vi "IonGuide.vi"() -> ()   [LabVIEW 2014, in "Panels.lvlib"]
uses:
  Panels.lvlib
  CSlibraries-extern/DimLVEvent/DimIndicators/DimIndicators.lvlib
  CSlibraries/UtilityLib/UtilityLib.lvlib
  CS_Core/CSSystem/CoreLib/CoreLib.lvlib
  CSlibraries/UtilityLib/UtilityLib.valueStatus.ctl
  CSlibraries-extern/DimLVEvent/LVDimInterface/LVDimInterface.lvlib
  Instance           1 16Saved   IonGuide .vi
  CS_Core/CSSystem/CoreLib/CoreLib.double 2 byte array.vi
  CS_Core/CSSystem/CoreLib/CoreLib.string 2 byte array.vi
  CS_Core/CSSystem/CoreLib/CoreLib.short 2 byte array.vi
  CSlibraries-extern/DimLVEvent/DimIndicators/DimIndicators.numericType.ctl
  CS_Core/BaseProcess/BaseProcess.descriptor string definition.ctl
  CS_Core/BaseProcess/BaseProcess.lvlib
  CS_Core/CSSystem/CoreDefs/CoreDefs.rawDataType.ctl
  CS_Core/CSSystem/CoreDefs/CoreDefs.call_type.ctl
  CSlibraries-extern/DimLVEvent/DimIndicators/DimIndicators.numericArrayType.ctl
  CSlibraries-extern/DimLVEvent/DimIndicators/DimIndicators.anyType.ctl
panel:
  in  "ListOfBases_Data":T1={"data"="NOLINK", "no link"=TRUE, "quality"=-1, "timeStamp"=0.0}
  in  "DC8_SetValueInfoData":T2={"data"=[-118.7, 118.8, 3.0], "no link"=FALSE, "quality"=0, "timeStamp"=3265900746.569}
  in  "DC7_SetValueInfoData":T2={"data"=[-118.7, 118.8, 3.0], "no link"=FALSE, "quality"=0, "timeStamp"=3265900746.569}
  in  "DC6_SetValueInfoData":T2={"data"=[-118.7, 118.8, 3.0], "no link"=FALSE, "quality"=0, "timeStamp"=3265900746.569}
  in  "DC8_SetData":T2={"data"=[0.0, 0.0, 0.0, 0.0], "no link"=FALSE, "quality"=1, "timeStamp"=3265900745.1}
  in  "DC6_SetData":T2={"data"=[0.0, 0.0, 0.0, 0.0], "no link"=FALSE, "quality"=1, "timeStamp"=3265900745.335}
  in  "DC7_SetData":T2={"data"=[0.0, 0.0, 0.0, 0.0], "no link"=FALSE, "quality"=1, "timeStamp"=3265900745.1}
  in  "DC8":bool
  in  "DC6":bool
  in  "DC7":bool
  in  "Offset_SetValueInfoData":T2={"data"=[-400.0, 400.0, 3.0], "no link"=FALSE, "quality"=0, "timeStamp"=3265900746.522}
  in  "Mass_SetData":T2={"data"=[0.0, 0.0, 0.0, 0.0], "no link"=FALSE, "quality"=1, "timeStamp"=3265900745.1}
  in  "IonGuideBase_SetValueInfoData":T2={"data"=[-400.0, 400.0, 3.0], "no link"=FALSE, "quality"=0, "timeStamp"=3265900746.522}
  in  "SetFileLocation_Data":T1={"data"="NOLINK", "no link"=TRUE, "quality"=-1, "timeStamp"=0.0}
  out "error out":errorcluster
  out "vi reference":refnum<vi>
  in  "Alpha":bool
  out "Alpha_Mon":dbl=inf format="%.4f"
  in  "Offset":bool
  out "Offset_Mon":dbl=inf format="%.4f"
  in  "Mass":bool
  out "Mass_Mon":dbl=inf format="%.4f"
  in  "RFamp3":bool
  out "RFamp3_Mon":dbl=inf format="%.4f"
  in  "RFphase2":bool
  in  "RFphase1":bool
  in  "DC5":bool
  in  "DC4":bool
  in  "RFamp2":bool
  in  "uPlate2":bool
  in  "uDC1":bool
  in  "uDC2":bool
  in  "RFamp1":bool
  in  "IGADC2":bool
  in  "uPlate1":bool
  in  "IGADC3":bool
  in  "IGADC1":bool
  in  "Alpha_SetValueInfoData":T2={"data"=[-404.0, 401.8, 3.0], "no link"=FALSE, "quality"=0, "timeStamp"=3265900746.569}
  in  "Mass_SetValueInfoData":T2={"data"=[-404.0, 401.8, 3.0], "no link"=FALSE, "quality"=0, "timeStamp"=3265900746.569}
  in  "Offset_SetData":T2={"data"=[0.0, 0.0, 0.0, 0.0], "no link"=FALSE, "quality"=1, "timeStamp"=3265900745.053}
  in  "Alpha_SetData":T2={"data"=[0.0, 0.0, 0.0, 0.0], "no link"=FALSE, "quality"=1, "timeStamp"=3265900745.053}
  in  "Alpha_MonData":T3={"data"=inf, "no link"=FALSE, "quality"=1, "timeStamp"=3265900746.538}
  in  "Mass_MonData":T3={"data"=inf, "no link"=FALSE, "quality"=1, "timeStamp"=3265900746.569}
  in  "Offset_MonData":T3={"data"=inf, "no link"=FALSE, "quality"=1, "timeStamp"=3265900746.554}
  in  "DC5_SetValueInfoData":T2={"data"=[-400.0, 400.0, 3.0], "no link"=FALSE, "quality"=0, "timeStamp"=3265900746.522}
  in  "DC4_SetValueInfoData":T2={"data"=[-118.7, 118.8, 3.0], "no link"=FALSE, "quality"=0, "timeStamp"=3265900746.569}
  in  "uDC2_SetValueInfoData":T2={"data"=[-120.9, 120.5, 3.0], "no link"=FALSE, "quality"=0, "timeStamp"=3265900746.585}
  in  "uDC1_SetValueInfoData":T2={"data"=[-120.8, 120.3, 3.0], "no link"=FALSE, "quality"=0, "timeStamp"=3265900746.569}
  in  "RFamp3_SetData":T2={"data"=[0.0, 0.0, 0.0, 0.0], "no link"=FALSE, "quality"=1, "timeStamp"=3265900745.335}
  in  "RFphase2_SetData":T2={"data"=[0.0, 0.0, 0.0, 0.0], "no link"=FALSE, "quality"=1, "timeStamp"=3265900745.1}
  in  "RFphase1_SetData":T2={"data"=[0.0, 0.0, 0.0, 0.0], "no link"=FALSE, "quality"=1, "timeStamp"=3265900745.1}
  in  "DC5_SetData":T2={"data"=[0.0, 0.0, 0.0, 0.0], "no link"=FALSE, "quality"=1, "timeStamp"=3265900745.069}
  in  "DC8_MonData":T3={"data"=inf, "no link"=FALSE, "quality"=1, "timeStamp"=3265900746.538}
  in  "MFDC2_MonData":T3={"data"=inf, "no link"=FALSE, "quality"=1, "timeStamp"=3265900746.538}
  in  "MFDC1_MonData":T3={"data"=inf, "no link"=FALSE, "quality"=1, "timeStamp"=3265900746.522}
  in  "RFphase2_MonData":T3={"data"=inf, "no link"=FALSE, "quality"=1, "timeStamp"=3265900746.569}
  in  "RFphase1_MonData":T3={"data"=inf, "no link"=FALSE, "quality"=1, "timeStamp"=3265900746.554}
  in  "IGADC1_MonData":T3={"data"=inf, "no link"=FALSE, "quality"=1, "timeStamp"=3265900746.538}
  in  "RFamp1_MonData":T3={"data"=inf, "no link"=FALSE, "quality"=1, "timeStamp"=3265900746.569}
  in  "uPlate1_MonData":T3={"data"=inf, "no link"=FALSE, "quality"=1, "timeStamp"=3265900746.554}
  out "RFphase2_Mon":dbl=inf format="%.4f"
  out "RFphase1_Mon":dbl=inf format="%.4f"
  out "MFDC1_Mon":dbl=inf format="%.4f"
  out "MFDC2_Mon":dbl=inf format="%.4f"
  out "DC5_Mon":dbl=inf format="%.4f"
  out "DC7_Mon":dbl=inf format="%.4f"
  out "DC8_Mon":dbl=inf format="%.4f"
  out "DC6_Mon":dbl=inf format="%.4f"
  in  "uDC2_MonData":T3={"data"=inf, "no link"=FALSE, "quality"=1, "timeStamp"=3265900746.538}
  in  "IGADC2_MonData":T3={"data"=inf, "no link"=FALSE, "quality"=1, "timeStamp"=3265900746.569}
  out "IGBPEN_Mon":dbl=inf format="%.2e"
  out "IGCPEN_Mon":dbl=inf format="%.2e"
  in  "uPlate2_SetValueInfoData":T2={"data"=[-125.5, 126.0, 3.0], "no link"=FALSE, "quality"=0, "timeStamp"=3265900746.554}
  in  "DC4_SetData":T2={"data"=[0.0, 0.0, 0.0, 0.0], "no link"=FALSE, "quality"=1, "timeStamp"=3265900745.069}
  in  "RFamp2_SetValueInfoData":T2={"data"=[0.0, 400.0, -1.0], "no link"=FALSE, "quality"=0, "timeStamp"=3265900746.585}
  in  "uPlate2_SetData":T2={"data"=[0.0, 0.0, 0.0, 0.0], "no link"=FALSE, "quality"=1, "timeStamp"=3265900745.069}
  in  "DC7_MonData":T3={"data"=inf, "no link"=FALSE, "quality"=1, "timeStamp"=3265900746.569}
  out "RFamp1_Mon":dbl=inf format="%.4f"
  out "IGADC1_Mon":dbl=inf format="%.4f"
  out "i ref out":refnum<vi>
  in  "Last Loaded File_Data":T1={"data"="NOLINK", "no link"=TRUE, "quality"=-1, "timeStamp"=0.0}
  out "FileUpToDate":bool=TRUE caption="Parameter Changed"
  in  "Close All Panels":bool
  in  "IGADC1_SetValueInfoData":T2={"data"=[-401.3, 400.4, 3.0], "no link"=FALSE, "quality"=0, "timeStamp"=3265900746.554}
  in  "IGADC2_SetValueInfoData":T2={"data"=[-404.3, 403.0, 3.0], "no link"=FALSE, "quality"=0, "timeStamp"=3265900746.538}
  in  "IGADC3_SetValueInfoData":T2={"data"=[-400.3, 399.3, 3.0], "no link"=FALSE, "quality"=0, "timeStamp"=3265900746.569}
  in  "RFamp3_SetValueInfoData":T2={"data"=[0.0, 3000.0, -1.0], "no link"=FALSE, "quality"=0, "timeStamp"=3265900746.554}
  in  "RFphase1_SetValueInfoData":T2={"data"=[0.0, 10.0, -1.0], "no link"=FALSE, "quality"=0, "timeStamp"=3265900746.522}
  in  "RFphase2_SetValueInfoData":T2={"data"=[0.0, 10.0, -1.0], "no link"=FALSE, "quality"=0, "timeStamp"=3265900746.538}
  in  "RFamp1_SetValueInfoData":T2={"data"=[0.0, 1000.0, -1.0], "no link"=FALSE, "quality"=0, "timeStamp"=3265900746.538}
  in  "uPlate1_SetValueInfoData":T2={"data"=[-404.0, 401.8, 3.0], "no link"=FALSE, "quality"=0, "timeStamp"=3265900746.569}
  in  "IonGuideBase_SetData":T2={"data"=[0.0, 0.0, 0.0, 0.0], "no link"=FALSE, "quality"=1, "timeStamp"=3265900745.1}
  in  "uDC1_SetData":T2={"data"=[0.0, 0.0, 0.0, 0.0], "no link"=FALSE, "quality"=1, "timeStamp"=3265900745.069}
  in  "IGADC3_SetData":T2={"data"=[0.0, 0.0, 0.0, 0.0], "no link"=FALSE, "quality"=1, "timeStamp"=3265900745.053}
  in  "IGADC2_SetData":T2={"data"=[0.0, 0.0, 0.0, 0.0], "no link"=FALSE, "quality"=1, "timeStamp"=3265900745.053}
  in  "IGADC1_SetData":T2={"data"=[0.0, 0.0, 0.0, 0.0], "no link"=FALSE, "quality"=1, "timeStamp"=3265900745.038}
  in  "RFamp2_SetData":T2={"data"=[0.0, 0.0, 0.0, 0.0], "no link"=FALSE, "quality"=1, "timeStamp"=3265900745.085}
  in  "RFamp1_SetData":T2={"data"=[0.0, 0.0, 0.0, 0.0], "no link"=FALSE, "quality"=1, "timeStamp"=3265900745.085}
  in  "uPlate1_SetData":T2={"data"=[0.0, 0.0, 0.0, 0.0], "no link"=FALSE, "quality"=1, "timeStamp"=3265900745.053}
  in  "uDC2_SetData":T2={"data"=[0.0, 0.0, 0.0, 0.0], "no link"=FALSE, "quality"=1, "timeStamp"=3265900745.069}
  in  "call cluster in":T4={"Object"="", "Selector"="", "CallType"=enum."synchronous", "Async Object"="", "Async Selector"="", "Data Descriptor"="", "Data"=[], "Error #"=0, "Expire"=0}
  in  "IonGuideBase":dbl
  out "Last Loaded File":string
  in  "SetFileLocation":path=path "\\\\intranet\\Files/projects/lebit/Data Exchange/data/IonGuideControl"
  in  "DC6_MonData":T3={"data"=inf, "no link"=FALSE, "quality"=1, "timeStamp"=3265900746.538}
  in  "DC5_MonData":T3={"data"=inf, "no link"=FALSE, "quality"=1, "timeStamp"=3265900746.585}
  in  "IGBPEN_MonData":T3={"data"=inf, "no link"=FALSE, "quality"=1, "timeStamp"=3265900746.538}
  in  "IGCPEN_MonData":T3={"data"=inf, "no link"=FALSE, "quality"=1, "timeStamp"=3265900746.554}
  in  "DC4_MonData":T3={"data"=inf, "no link"=FALSE, "quality"=1, "timeStamp"=3265900746.569}
  in  "IGADC3_MonData":T3={"data"=inf, "no link"=FALSE, "quality"=1, "timeStamp"=3265900746.522}
  in  "RFamp3_MonData":T3={"data"=inf, "no link"=FALSE, "quality"=1, "timeStamp"=3265900746.538}
  in  "RFamp2_MonData":T3={"data"=inf, "no link"=FALSE, "quality"=1, "timeStamp"=3265900746.6}
  in  "uPlate2_MonData":T3={"data"=inf, "no link"=FALSE, "quality"=1, "timeStamp"=3265900746.585}
  in  "uDC1_MonData":T3={"data"=inf, "no link"=FALSE, "quality"=1, "timeStamp"=3265900746.569}
  out "DC4_Mon":dbl=inf format="%.4f"
  out "uPlate2_Mon":dbl=inf format="%.4f"
  out "IGADC2_Mon":dbl=inf format="%.4f"
  out "RFamp2_Mon":dbl=inf format="%.4f"
  out "uDC1_Mon":dbl=inf format="%.4f"
  out "IGADC3_Mon":dbl=inf format="%.4f"
  out "uDC2_Mon":dbl=inf format="%.4f"
  out "uPlate1_Mon":dbl=inf format="%.4f"
  # "Parameter changed, data file is no longer up-to-date."
  # "IGBPEN"
  # "IGCPEN"
  # "Values in italic don't have a real monitor"
  # "MFDC1"
  # "MFDC2"
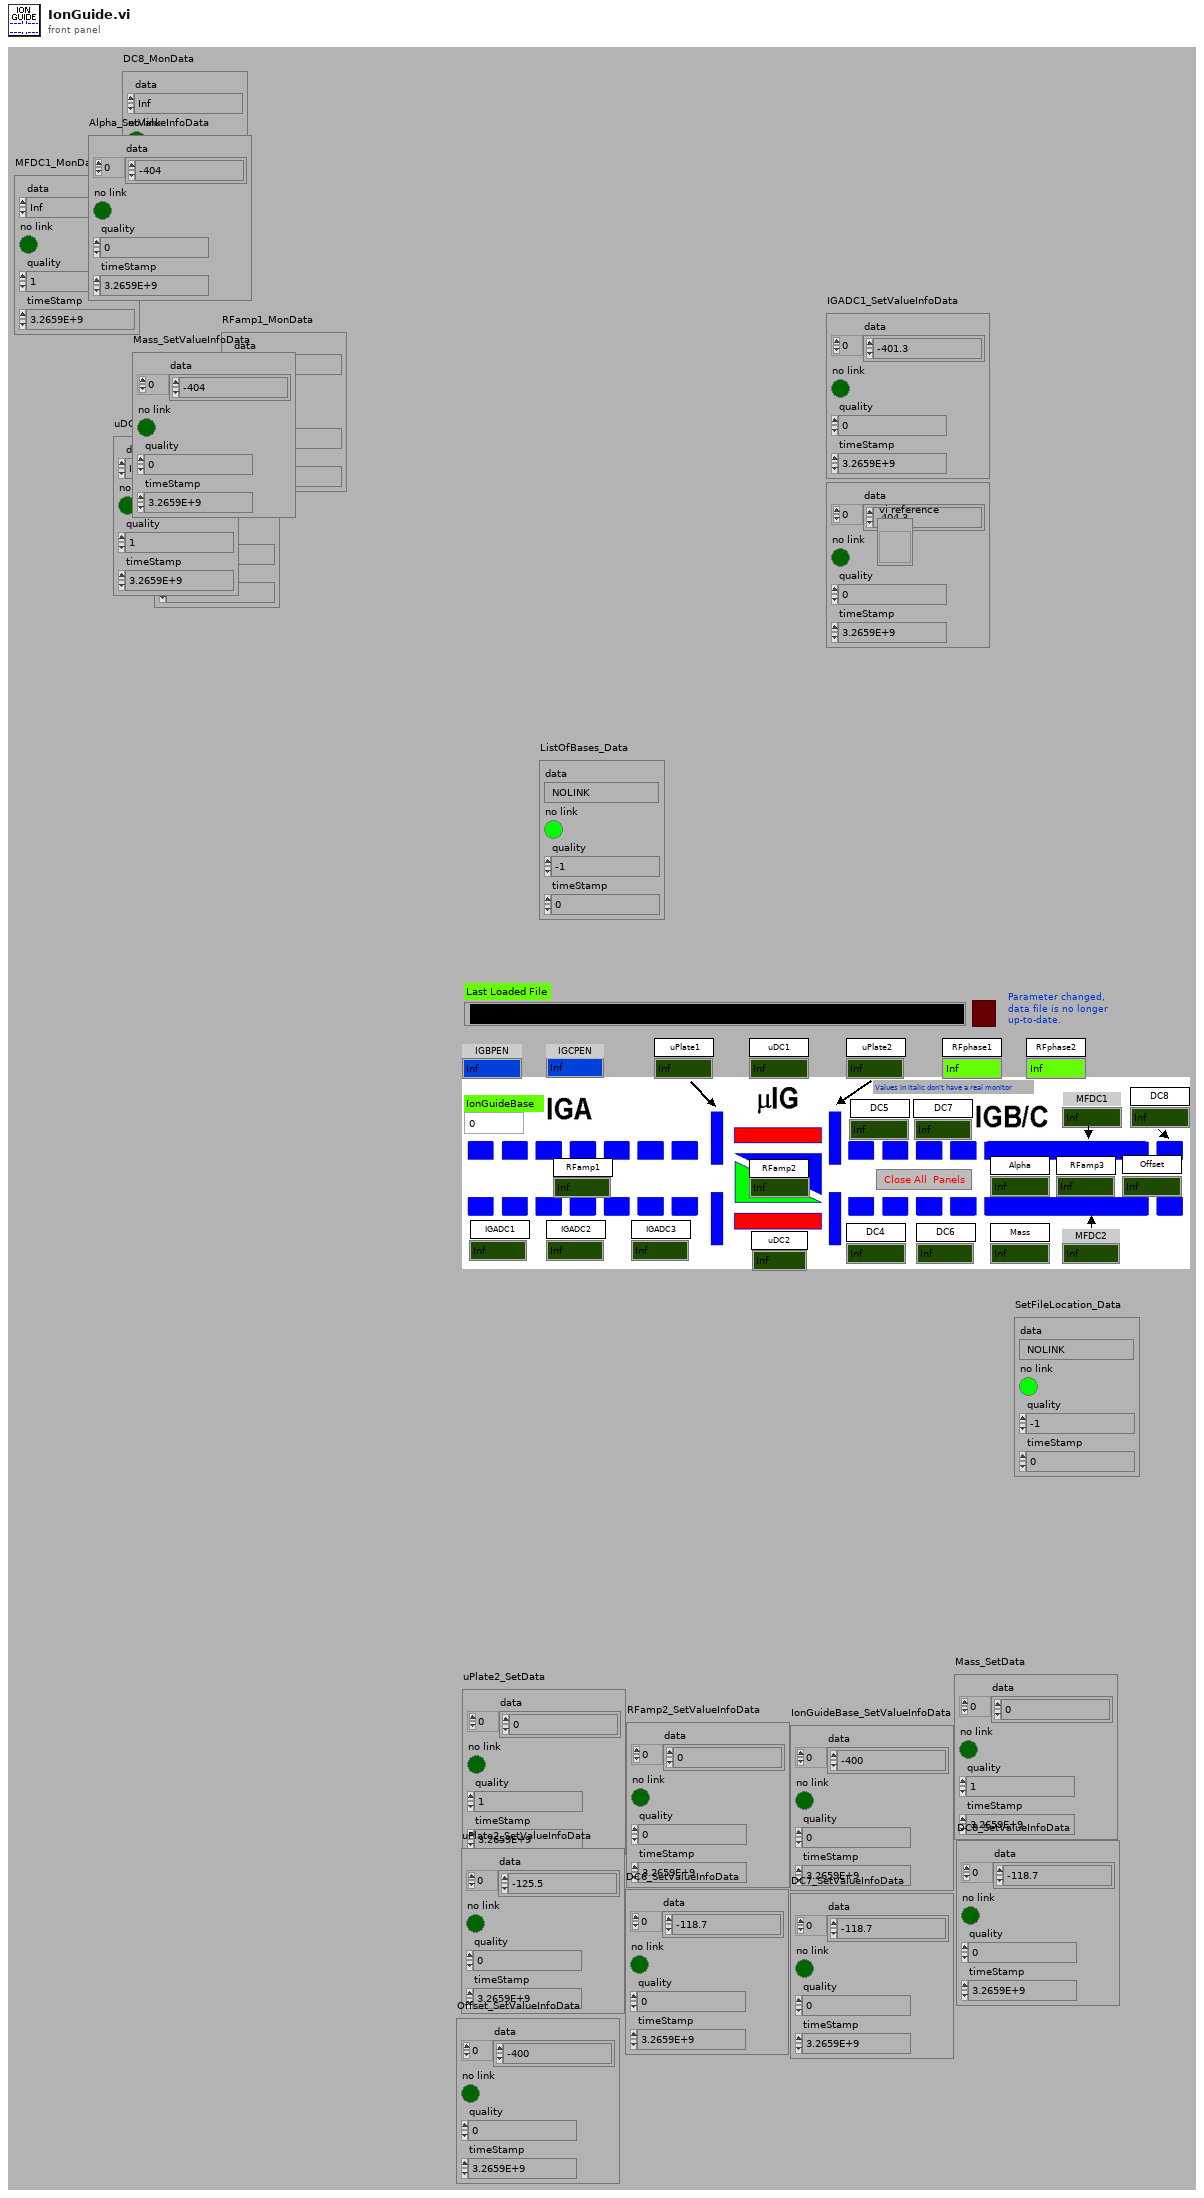
[diagram p1: front panel]
types:
  T1 = typedef "DimIndicators.lvlib/DimIndicators.anyType.ctl" = cluster{"data":string, "no link":bool, "quality":i32, "timeStamp":dbl}
  T2 = typedef "DimIndicators.lvlib/DimIndicators.numericArrayType.ctl" = cluster{"data":dbl[], "no link":bool, "quality":i32, "timeStamp":dbl}
  T3 = typedef "DimIndicators.lvlib/DimIndicators.numericType.ctl" = cluster{"data":dbl, "no link":bool, "quality":i32, "timeStamp":dbl}
  T4 = typedef "CoreDefs.call_type.ctl" = cluster{"Object":string, "Selector":string, "CallType":enum16{"simple", "synchronous", "asynchronous"}, "Async Object":string, "Async Selector":string, "Data Descriptor":T5, "Data":T6, "Error #":i32, "Expire":u32}
  T5 = typedef "BaseProcess.lvlib/BaseProcess.descriptor string definition.ctl" = string
  T6 = typedef "CoreDefs.rawDataType.ctl" = i8[]
  T7 = typedef "UtilityLib.lvlib/UtilityLib.valueStatus.ctl" = enum16{"no info available", "stand by/off", "on", "warning", "alarm/malfunction", "not implemented", "user action required", "important information", "system default", "control default", "indicator default", "button default"}
  T8 = cluster{"data":string, "no link":bool, "quality":i32, "timeStamp":dbl}
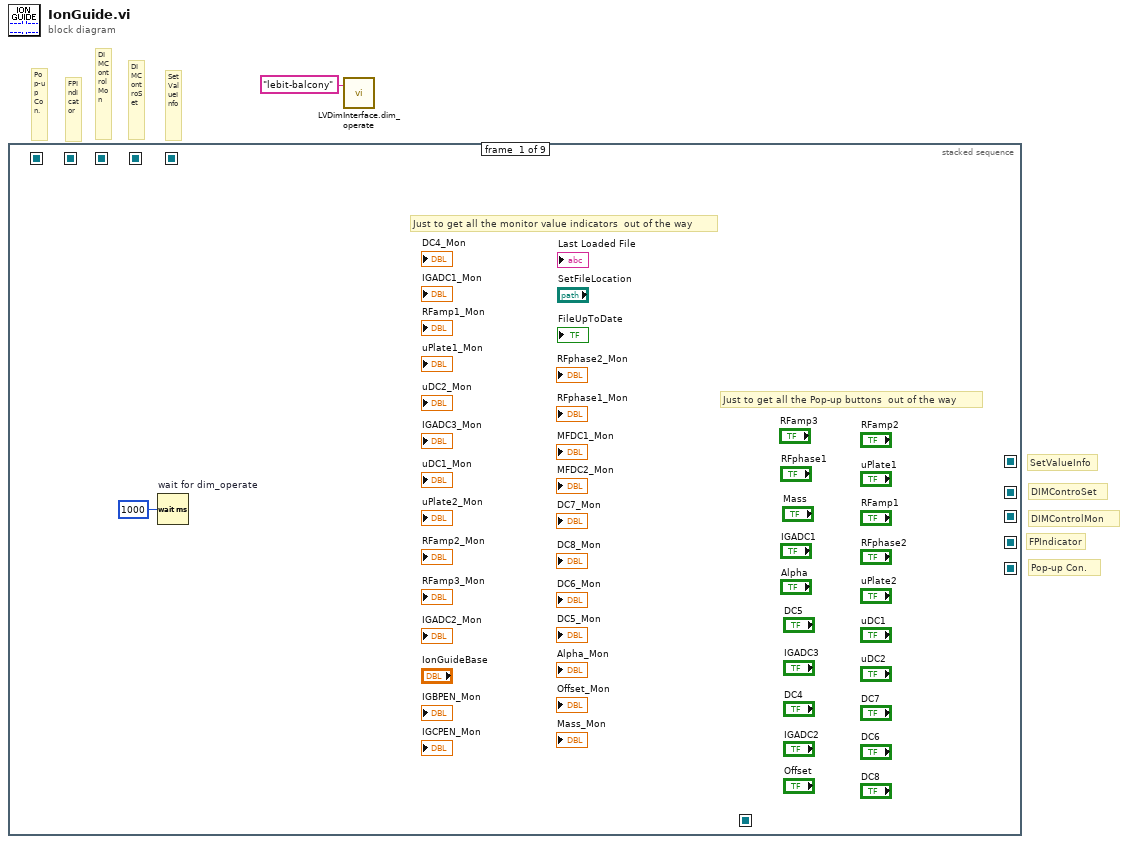
[diagram p0: block diagram]
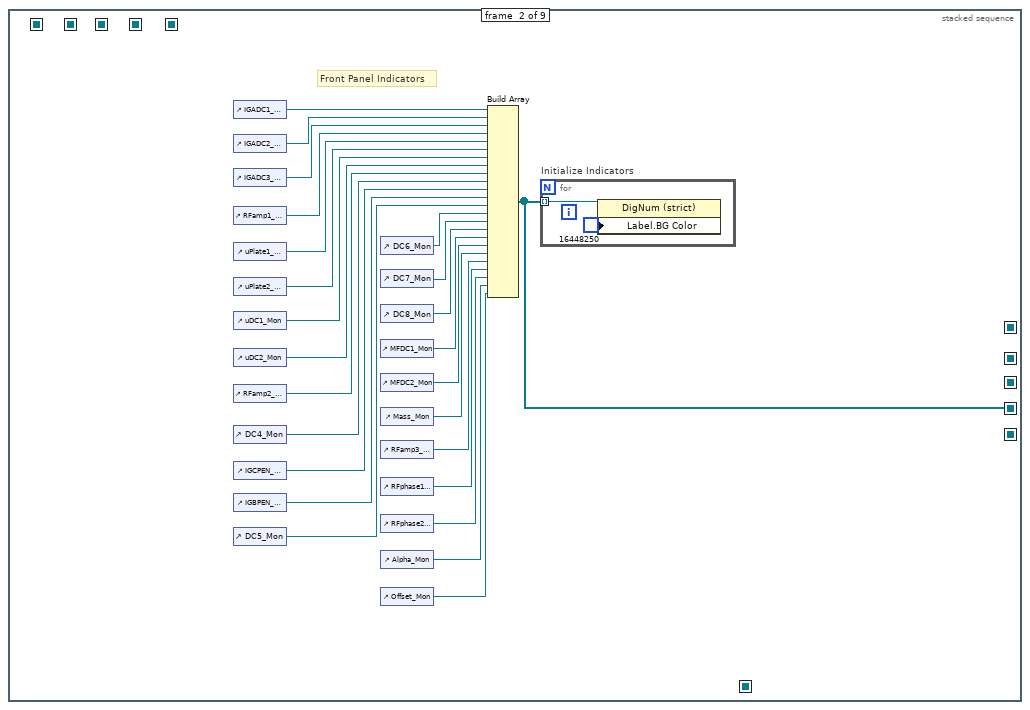
[diagram p2: hidden frame]
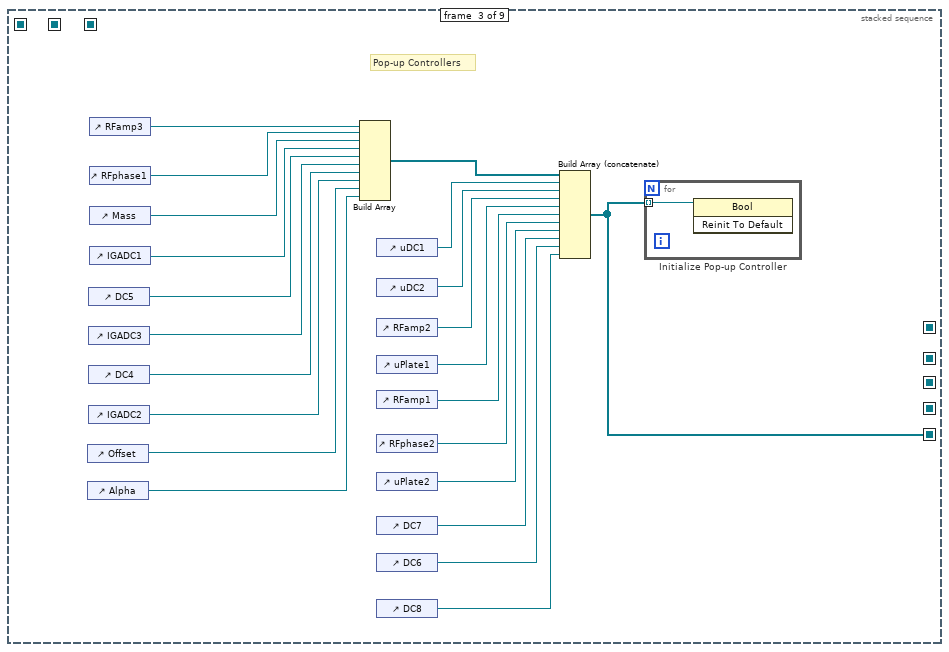
[diagram p3: hidden frame]
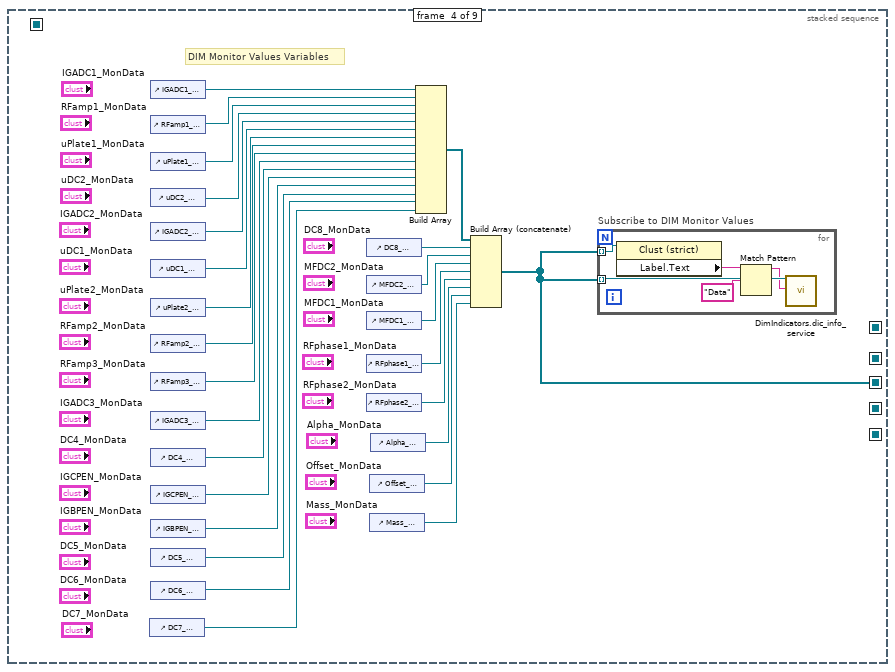
[diagram p4: hidden frame]
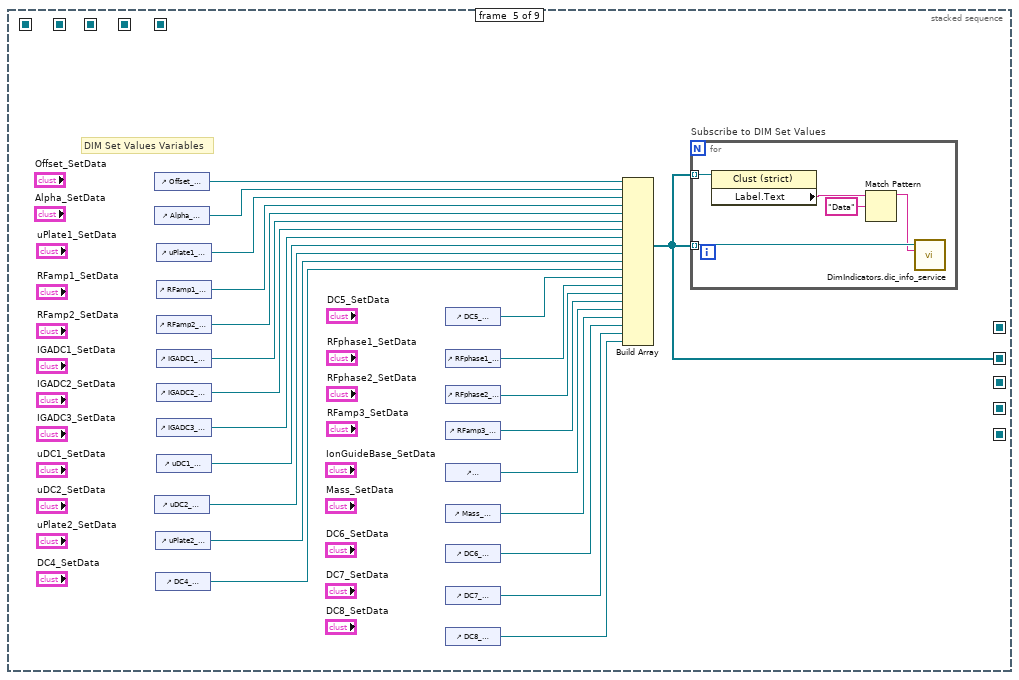
[diagram p5: hidden frame]
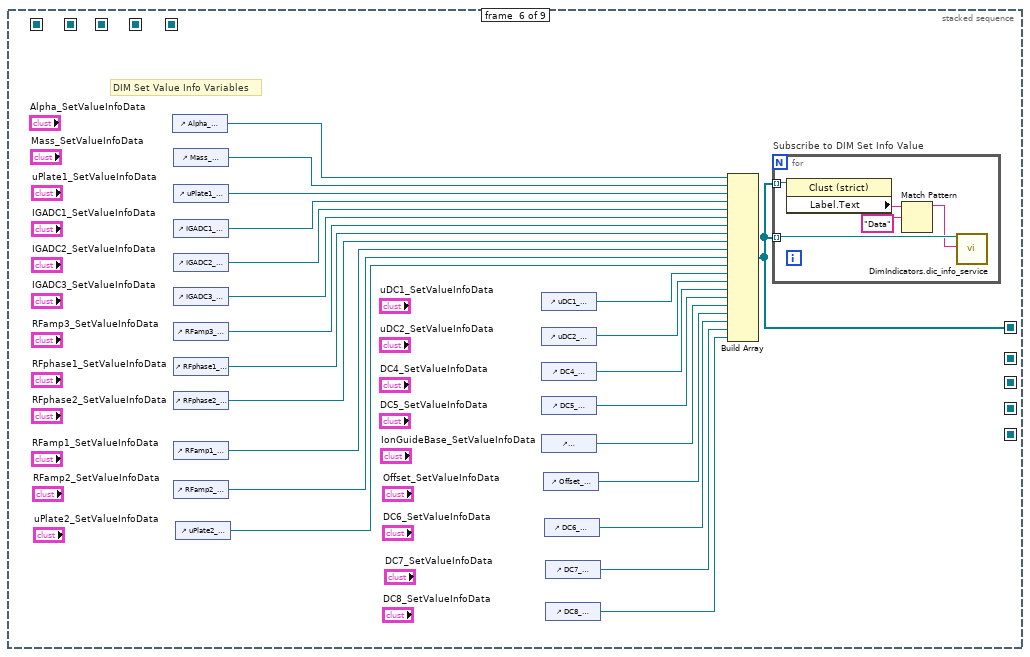
[diagram p6: hidden frame]
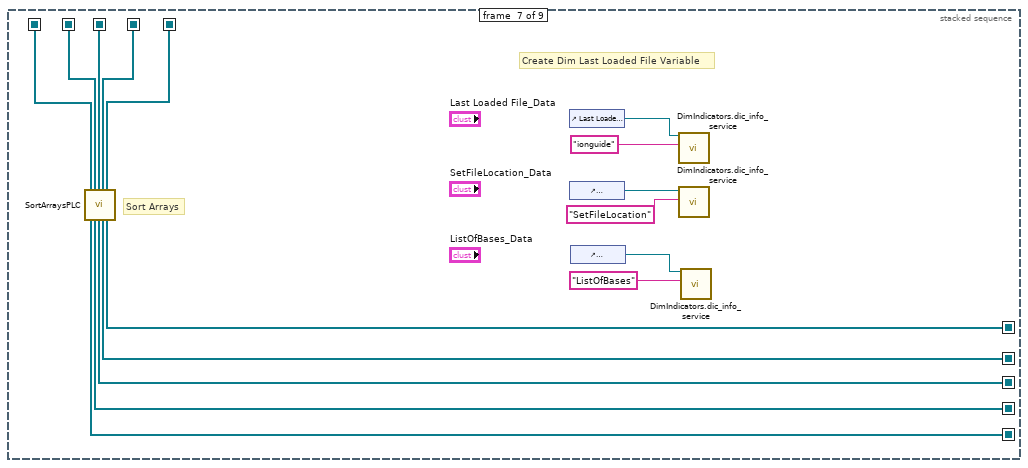
[diagram p7: hidden frame]
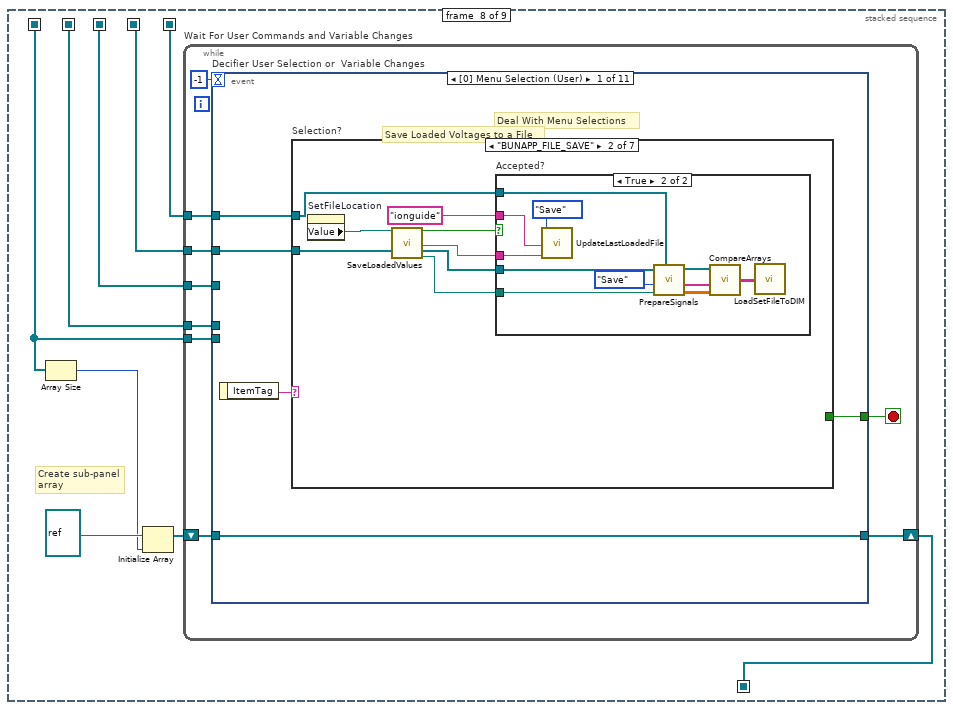
[diagram p8: hidden frame]
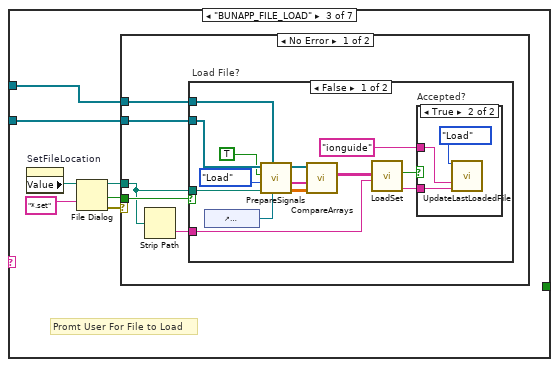
[diagram p11: hidden frame]
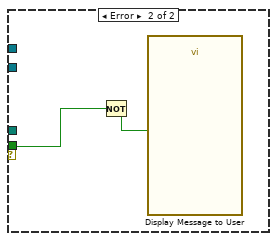
[diagram p14: hidden frame]
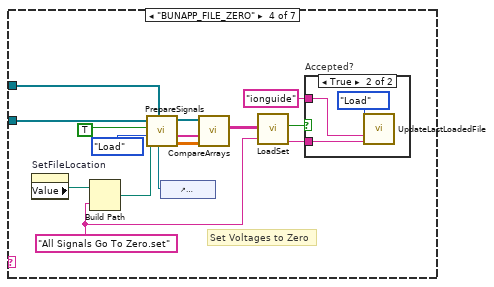
[diagram p15: hidden frame]
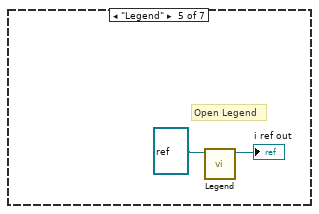
[diagram p17: hidden frame]
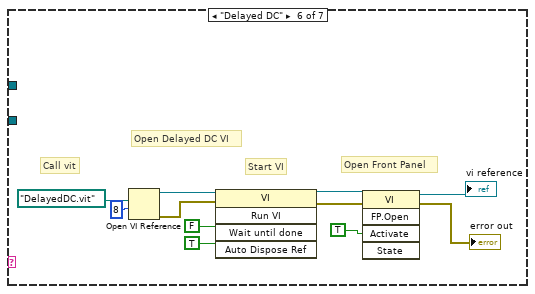
[diagram p18: hidden frame]
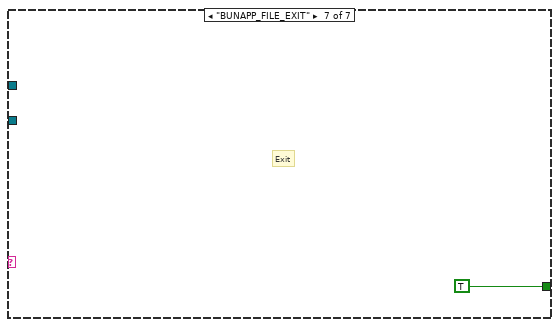
[diagram p19: hidden frame]
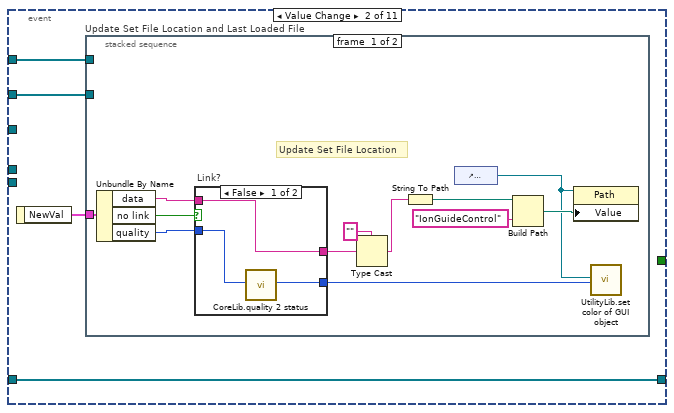
[diagram p20: hidden frame]
diagram:
  # "DIMControlMon"
  # "DIMControSet"
  # "SetValueInfo"
  # "Pop-up Con."
  # "FPIndicator"
  # "Pop-up Con."
  # "SetValueInfo"
  # "DIMControSet"
  # "DIMControlMon"
  # "FPIndicator"
  n1 = stacked-sequence {
    seq-local: [_ _ _ _ _ _ w150 _ _] -> [_ _ _ _ _ _ _ w159 _]
    seq-local: [_ _ _ _ _ _ w151 _ _] -> [_ _ _ _ _ _ _ w162 w414]
    seq-local: [_ _ _ _ _ _ _ w157 _] -> [_ _ _ _ _ _ _ _ w413]
    seq-local: [_ _ _ _ _ _ w152 _ _] -> [_ _ _ _ _ _ _ w156 w412]
    seq-local: [_ _ _ _ _ _ w153 _ _] -> [_ _ _ _ _ _ _ w155 w411]
    seq-local: [_ _ _ _ _ _ w149 _ _] -> [_ _ _ _ _ _ _ w154 _]
    seq-local: [_ w4 _ _ _ _ _ _ _] -> [_ _ _ _ _ _ w145 _ _]
    seq-local: [_ _ w34 _ _ _ _ _ _] -> [_ _ _ _ _ _ w144 _ _]
    seq-local: [_ _ _ w53 _ _ _ _ _] -> [_ _ _ _ _ _ w146 _ _]
    seq-local: [_ _ _ _ w88 _ _ _ _] -> [_ _ _ _ _ _ w147 _ _]
    seq-local: [_ _ _ _ _ w116 _ _ _] -> [_ _ _ _ _ _ w148 _ _]
    frame #0 {
      # "Just to get all the Pop-up buttons  out of the way"
      # "Just to get all the monitor value indicators  out of the way"
      n2 = Wait (ms) "wait for dim_operate"(milliseconds to wait=u32 1000) -> ()  [unwired: 1 out]
    }
    frame #1 {
      # "Front Panel Indicators"
      # "Arrange references to all monitor-value related buttons into an array."
      n3 = control-ref of="IGADC1_Mon"() -> (w26:refnum<vi>)
      n4 = control-ref of="IGADC2_Mon"() -> (w14:refnum<vi>)
      n5 = control-ref of="IGADC3_Mon"() -> (w13:refnum<vi>)
      n6 = control-ref of="RFamp1_Mon"() -> (w12:refnum<vi>)
      n7 = control-ref of="uPlate1_Mon"() -> (w11:refnum<vi>)
      n8 = control-ref of="uPlate2_Mon"() -> (w27:refnum<vi>)
      n9 = control-ref of="uDC1_Mon"() -> (w10:refnum<vi>)
      n10 = control-ref of="uDC2_Mon"() -> (w9:refnum<vi>)
      n11 = control-ref of="RFamp2_Mon"() -> (w8:refnum<vi>)
      n12 = control-ref of="DC4_Mon"() -> (w25:refnum<vi>)
      n13 = control-ref of="IGCPEN_Mon"() -> (w24:refnum<vi>)
      n14 = control-ref of="IGBPEN_Mon"() -> (w23:refnum<vi>)
      n15 = control-ref of="DC5_Mon"() -> (w22:refnum<vi>)
      n16 = control-ref of="DC6_Mon"() -> (w17:refnum<vi>)
      n17 = control-ref of="DC7_Mon"() -> (w21:refnum<vi>)
      n18 = control-ref of="DC8_Mon"() -> (w20:refnum<vi>)
      n19 = control-ref of="MFDC1_Mon"() -> (w7:refnum<vi>)
      n20 = control-ref of="MFDC2_Mon"() -> (w6:refnum<vi>)
      n21 = control-ref of="Mass_Mon"() -> (w3:refnum<vi>)
      n22 = control-ref of="RFamp3_Mon"() -> (w5:refnum<vi>)
      n23 = control-ref of="RFphase1_Mon"() -> (w19:refnum<vi>)
      n24 = control-ref of="RFphase2_Mon"() -> (w18:refnum<vi>)
      n25 = control-ref of="Alpha_Mon"() -> (w16:refnum<vi>)
      n26 = control-ref of="Offset_Mon"() -> (w15:refnum<vi>)
      n27 = Build Array(w26, w14, w13, w12, w11, w27, w10, w9, w8, w25, w24, w23, w22, w17, w21, w20, w7, w6, w3, w5, w19, w18, w16, w15) -> (w4:refnum<vi>[])
      n28 = for "Initialize Indicators" {
        tunnel: w4 -> [w29] mode=indexing
        n29 = property class="DigNum (strict)"(reference=w29, "Label.BG Color"=u32 16448250 ("Color Box")) -> ()  [unwired: 1 in, 2 out]
      }
    }
    frame #2 {
      # "Pop-up Controllers"
      n30 = control-ref of="Offset"() -> (w44:refnum<vi>)
      n31 = control-ref of="Alpha"() -> (w43:refnum<vi>)
      n32 = control-ref of="DC5"() -> (w48:refnum<vi>)
      n33 = control-ref of="IGADC3"() -> (w47:refnum<vi>)
      n34 = control-ref of="DC4"() -> (w46:refnum<vi>)
      n35 = control-ref of="IGADC2"() -> (w45:refnum<vi>)
      n36 = control-ref of="RFamp3"() -> (w51:refnum<vi>)
      n37 = control-ref of="RFphase1"() -> (w50:refnum<vi>)
      n38 = control-ref of="Mass"() -> (w33:refnum<vi>)
      n39 = control-ref of="IGADC1"() -> (w49:refnum<vi>)
      n40 = Build Array(w51, w50, w33, w49, w48, w47, w46, w45, w44, w43) -> (w42:refnum<vi>[])
      n41 = control-ref of="uDC1"() -> (w41:refnum<vi>)
      n42 = control-ref of="uDC2"() -> (w40:refnum<vi>)
      n43 = control-ref of="RFamp2"() -> (w39:refnum<vi>)
      n44 = control-ref of="uPlate1"() -> (w38:refnum<vi>)
      n45 = control-ref of="RFamp1"() -> (w37:refnum<vi>)
      n46 = control-ref of="RFphase2"() -> (w36:refnum<vi>)
      n47 = control-ref of="uPlate2"() -> (w35:refnum<vi>)
      n48 = control-ref of="DC7"() -> (w32:refnum<vi>)
      n49 = control-ref of="DC6"() -> (w31:refnum<vi>)
      n50 = control-ref of="DC8"() -> (w30:refnum<vi>)
      n51 = Build Array (concatenate)(w42, w41, w40, w39, w38, w37, w36, w35, w32, w31, w30) -> (w34:refnum<vi>[])
      n52 = for "Initialize Pop-up Controller" {
        tunnel: w34 -> [w52] mode=indexing
        n53 = invoke class="Bool" method="Reinit To Default"(reference=w52) -> ()  [unwired: 2 in, 3 out]
      }
    }
    frame #3 {
      # "DIM Monitor Values Variables"
      n54 = control-ref of="DC7_MonData"() -> (w58:refnum<vi>)
      n55 = control-ref of="IGADC1_MonData"() -> (w63:refnum<vi>)
      n56 = control-ref of="RFamp1_MonData"() -> (w64:refnum<vi>)
      n57 = control-ref of="uPlate1_MonData"() -> (w65:refnum<vi>)
      n58 = control-ref of="uDC2_MonData"() -> (w70:refnum<vi>)
      n59 = control-ref of="IGADC2_MonData"() -> (w69:refnum<vi>)
      n60 = control-ref of="uDC1_MonData"() -> (w78:refnum<vi>)
      n61 = control-ref of="uPlate2_MonData"() -> (w77:refnum<vi>)
      n62 = control-ref of="RFamp2_MonData"() -> (w76:refnum<vi>)
      n63 = control-ref of="RFamp3_MonData"() -> (w75:refnum<vi>)
      n64 = control-ref of="IGADC3_MonData"() -> (w74:refnum<vi>)
      n65 = control-ref of="DC4_MonData"() -> (w73:refnum<vi>)
      n66 = control-ref of="IGCPEN_MonData"() -> (w72:refnum<vi>)
      n67 = control-ref of="IGBPEN_MonData"() -> (w71:refnum<vi>)
      n68 = control-ref of="DC5_MonData"() -> (w60:refnum<vi>)
      n69 = control-ref of="DC6_MonData"() -> (w59:refnum<vi>)
      n70 = control-ref of="DC8_MonData"() -> (w68:refnum<vi>)
      n71 = control-ref of="MFDC2_MonData"() -> (w67:refnum<vi>)
      n72 = control-ref of="MFDC1_MonData"() -> (w66:refnum<vi>)
      n73 = control-ref of="RFphase1_MonData"() -> (w62:refnum<vi>)
      n74 = control-ref of="RFphase2_MonData"() -> (w61:refnum<vi>)
      n75 = control-ref of="Offset_MonData"() -> (w55:refnum<vi>)
      n76 = control-ref of="Mass_MonData"() -> (w54:refnum<vi>)
      n77 = control-ref of="Alpha_MonData"() -> (w56:refnum<vi>)
      n78 = Build Array(w63, w64, w65, w70, w69, w78, w77, w76, w75, w74, w73, w72, w71, w60, w59, w58) -> (w57:refnum<vi>[])
      n79 = Build Array (concatenate)(w57, w68, w67, w66, w62, w61, w56, w55, w54) -> (w53:refnum<vi>[])
      n80 = for "Subscribe to DIM Monitor Values" {
        tunnel: w53 -> [w83] mode=indexing
        tunnel: w53 -> [w82] mode=indexing
        n81 = property class="Clust (strict)"(reference=w83) -> ("Label.Text"=w81:string)  [unwired: 1 in, 2 out]
        n82 = Match Pattern(string=w81, regular expression="Data") -> (before substring=w80:string)  [unwired: 1 in, 3 out]
        n83 = call "DimIndicators.dic_info_service.vi"("controlRef"=w82, "serviceName"=w80) -> ()  [unwired: 16 in, 2 out]
      }
    }
    frame #4 {
      # "DIM Set Values Variables"
      n84 = control-ref of="Offset_SetData"() -> (w89:refnum<vi>)
      n85 = control-ref of="Alpha_SetData"() -> (w90:refnum<vi>)
      n86 = control-ref of="uDC2_SetData"() -> (w98:refnum<vi>)
      n87 = control-ref of="uPlate2_SetData"() -> (w97:refnum<vi>)
      n88 = control-ref of="DC4_SetData"() -> (w96:refnum<vi>)
      n89 = control-ref of="uPlate1_SetData"() -> (w105:refnum<vi>)
      n90 = control-ref of="RFamp1_SetData"() -> (w104:refnum<vi>)
      n91 = control-ref of="RFamp2_SetData"() -> (w103:refnum<vi>)
      n92 = control-ref of="IGADC1_SetData"() -> (w102:refnum<vi>)
      n93 = control-ref of="IGADC2_SetData"() -> (w101:refnum<vi>)
      n94 = control-ref of="IGADC3_SetData"() -> (w100:refnum<vi>)
      n95 = control-ref of="uDC1_SetData"() -> (w99:refnum<vi>)
      n96 = control-ref of="DC5_SetData"() -> (w95:refnum<vi>)
      n97 = control-ref of="RFphase1_SetData"() -> (w94:refnum<vi>)
      n98 = control-ref of="RFphase2_SetData"() -> (w93:refnum<vi>)
      n99 = control-ref of="RFamp3_SetData"() -> (w92:refnum<vi>)
      n100 = control-ref of="IonGuideBase_SetData"() -> (w91:refnum<vi>)
      n101 = control-ref of="Mass_SetData"() -> (w87:refnum<vi>)
      n102 = control-ref of="DC6_SetData"() -> (w86:refnum<vi>)
      n103 = control-ref of="DC7_SetData"() -> (w85:refnum<vi>)
      n104 = control-ref of="DC8_SetData"() -> (w84:refnum<vi>)
      n105 = Build Array(w89, w90, w105, w104, w103, w102, w101, w100, w99, w98, w97, w96, w95, w94, w93, w92, w91, w87, w86, w85, w84) -> (w88:refnum<vi>[])
      n106 = for "Subscribe to DIM Set Values" {
        tunnel: w88 -> [w106] mode=indexing
        tunnel: w88 -> [w110] mode=indexing
        n107 = property class="Clust (strict)"(reference=w106) -> ("Label.Text"=w109:string)  [unwired: 1 in, 2 out]
        n108 = Match Pattern(string=w109, regular expression="Data") -> (before substring=w107:string)  [unwired: 1 in, 3 out]
        n109 = call "DimIndicators.dic_info_service.vi"("controlRef"=w110, "serviceName"=w107) -> ()  [unwired: 16 in, 2 out]
      }
    }
    frame #5 {
      # "DIM Set Value Info Variables"
      n110 = control-ref of="Alpha_SetValueInfoData"() -> (w118:refnum<vi>)
      n111 = control-ref of="Mass_SetValueInfoData"() -> (w117:refnum<vi>)
      n112 = control-ref of="uPlate1_SetValueInfoData"() -> (w132:refnum<vi>)
      n113 = control-ref of="IGADC1_SetValueInfoData"() -> (w131:refnum<vi>)
      n114 = control-ref of="IGADC2_SetValueInfoData"() -> (w130:refnum<vi>)
      n115 = control-ref of="IGADC3_SetValueInfoData"() -> (w129:refnum<vi>)
      n116 = control-ref of="RFamp3_SetValueInfoData"() -> (w128:refnum<vi>)
      n117 = control-ref of="RFphase1_SetValueInfoData"() -> (w127:refnum<vi>)
      n118 = control-ref of="RFphase2_SetValueInfoData"() -> (w126:refnum<vi>)
      n119 = control-ref of="RFamp1_SetValueInfoData"() -> (w125:refnum<vi>)
      n120 = control-ref of="RFamp2_SetValueInfoData"() -> (w124:refnum<vi>)
      n121 = control-ref of="uPlate2_SetValueInfoData"() -> (w123:refnum<vi>)
      n122 = control-ref of="uDC1_SetValueInfoData"() -> (w122:refnum<vi>)
      n123 = control-ref of="uDC2_SetValueInfoData"() -> (w121:refnum<vi>)
      n124 = control-ref of="DC4_SetValueInfoData"() -> (w120:refnum<vi>)
      n125 = control-ref of="DC5_SetValueInfoData"() -> (w119:refnum<vi>)
      n126 = control-ref of="IonGuideBase_SetValueInfoData"() -> (w115:refnum<vi>)
      n127 = control-ref of="Offset_SetValueInfoData"() -> (w114:refnum<vi>)
      n128 = control-ref of="DC6_SetValueInfoData"() -> (w113:refnum<vi>)
      n129 = control-ref of="DC7_SetValueInfoData"() -> (w112:refnum<vi>)
      n130 = control-ref of="DC8_SetValueInfoData"() -> (w111:refnum<vi>)
      n131 = Build Array(w118, w117, w132, w131, w130, w129, w128, w127, w126, w125, w124, w123, w122, w121, w120, w119, w115, w114, w113, w112, w111) -> (w116:refnum<vi>[])
      n132 = for "Subscribe to DIM Set Info Value" {
        tunnel: w116 -> [w133] mode=indexing
        tunnel: w116 -> [w137] mode=indexing
        n133 = property class="Clust (strict)"(reference=w133) -> ("Label.Text"=w136:string)  [unwired: 1 in, 2 out]
        n134 = Match Pattern(string=w136, regular expression="Data") -> (before substring=w134:string)  [unwired: 1 in, 3 out]
        n135 = call "DimIndicators.dic_info_service.vi"("controlRef"=w137, "serviceName"=w134) -> ()  [unwired: 16 in, 2 out]
      }
    }
    frame #6 {
      # "Create Dim Last Loaded File Variable"
      # "Sort Arrays"
      n136 = call "SortArraysPLC.vi"("Pop-up Con."=w144, "FPIndicator in"=w145, "DIMControlMon"=w146, "DIMControSet"=w147, "SetValueInfo"=w148) -> ("Pop-up Con. out"=w149:refnum<vi>[], "FPIndicator out"=w150:refnum<vi>[], "DIMControlMon out"=w151:refnum<vi>[], "DIMControSet out"=w152:refnum<vi>[], "SetValueInfo out"=w153:refnum<vi>[])  [unwired: 18 in]
      n137 = control-ref of="Last Loaded File_Data"() -> (w142:refnum<vi>)
      n138 = control-ref of="SetFileLocation_Data"() -> (w141:refnum<vi>)
      n139 = control-ref of="ListOfBases_Data"() -> (w139:refnum<vi>)
      n140 = call "DimIndicators.dic_info_service.vi"("controlRef"=w142, "serviceName"="ionguide" ("string")) -> ()  [unwired: 16 in, 2 out]
      n141 = call "DimIndicators.dic_info_service.vi"("controlRef"=w141, "serviceName"="SetFileLocation") -> ()  [unwired: 16 in, 2 out]
      n142 = call "DimIndicators.dic_info_service.vi"("controlRef"=w139, "serviceName"="ListOfBases" ("string")) -> ()  [unwired: 16 in, 2 out]
    }
    frame #7 {
      # "Create sub-panel\narray"
      n143 = Array Size(array=w154) -> (size(s)=w158:i32)
      n144 = Initialize Array(refnum<vi> refnum ("vi reference"), w158) -> (w161:refnum<vi>[])
      n145 = while "Wait For User Commands and Variable Changes" {
        tunnel: w162 -> [w170]
        tunnel: w159 -> [w169]
        shift-right: [w167] -> w157
        shift-left: w161 -> [w168]
        tunnel: w156 -> [w166]
        tunnel: w155 -> [w165]
        tunnel: w154 -> [w163]
        stop <- w171 stop-if-true
        n146 = event "Decifier User Selection or  Variable Changes" shown="[0] Menu Selection (User)" {
          selector: _ -> [_ _ _ _ _ _ _ _ _ _ _]
          dyn-events: _ -> [_ _ _ _ _ _ _ _ _ _ _]
          timeout: -1 -> [_ _ _ _ _ _ _ _ _ _ _]
          tunnel: [w173 _ _ _ _ _ _ _ _ _ TRUE ("stop")] -> w171
          tunnel: w170 -> [_ _ _ _ _ w343 _ _ _ _ w386]
          tunnel: w169 -> [_ _ _ _ _ w339 _ _ _ _ _]
          tunnel: w168 -> [w176 w260 w295 w302 w325 w345 w363 w371 w378 w384 w385]
          tunnel: [w176 w260 w295 w302 w325 w345 w363 w369 w376 w384 _] -> w167
          tunnel: w166 -> [w174 w261 w293 w303 w322 _ w361 _ _ _ w387]
          tunnel: w165 -> [w172 w259 w289 w304 _ _ _ _ _ _ w388]
          tunnel: w163 -> [_ _ _ _ _ _ _ w365 _ _ _]
          event Menu Selection (User) {
            # "Deal With Menu Selections"
            n147 = event-data() -> ("ItemTag"=w175:string)  [unwired: 1 in]
            n148 = case "Selection?" shown="\"BUNAPP_FILE_SAVE\"" w175 {
              tunnel: w174 -> [_ w181 w201 w241 _ _ _]
              tunnel: [_ _ _ _ _ _ TRUE ("stop")] -> w173
              tunnel: w172 -> [_ w177 w196 w228 _ _ _]
              frame "False", Default {
              }
              frame "BUNAPP_FILE_SAVE" {
                # "Save Loaded Voltages to a File"
                n149 = property on="SetFileLocation" class="Path"() -> ("Value"=w182:path)  [unwired: 2 in, 2 out]
                n150 = call "SaveLoadedValues.vi"("Panel Location?"=w182, "DIMControlSet in"=w181) -> ("File Saved?"=w183:bool, "File Name"=w180:string, "DIMControlSet out"=w178:refnum<vi>[], "Path"=w179:path)  [unwired: 14 in]
                n151 = case "Accepted?" shown="True" w183 {
                  tunnel: w180 -> [_ w193]
                  tunnel: "ionguide" ("string") -> [_ w195]
                  tunnel: w178 -> [_ w194]
                  tunnel: w179 -> [_ w192]
                  tunnel: w177 -> [_ w186]
                  frame False {
                  }
                  frame True {
                    n152 = call "UpdateLastLoadedFile.vi"("LoadOrSave"=enum16{"Load", "Save"}."Save", "GUIName"=w195, "FileNameIn"=w193) -> ()  [unwired: 13 in]
                    n153 = call "PrepareSignals.vi"("SetValueInfo in"=w186, "setfile path"=w192, "Enum"=enum16{"Save", "Load"}."Save", "DIMControSet in"=w194) -> ("indexed loaded Array"=w190:dbl[][], "Name Array"=w191:string[], "DIMControSet out"=w189:refnum<vi>[])  [unwired: 5 in]
                    n154 = call "CompareArrays.vi"("indexed loaded Array"=w190, "Name Array"=w191, "DIMControSet"=w189) -> ("Table for loading values"=w188:string[][])  [unwired: 4 in]
                    n155 = call "LoadSetFileToDIM.vi"("output array"=w188) -> ()  [unwired: 2 in]
                  }
                }
              }
              frame "BUNAPP_FILE_LOAD" {
                # "Promt User For File to Load"
                n156 = property on="SetFileLocation" class="Path"() -> ("Value"=w198:path)  [unwired: 2 in, 2 out]
                n157 = File Dialog(6:"*.set" ("pattern (all files)"), 11:w198) -> (0:w197:errorcluster, 1:w202:bool, 3:w199:path)  [unwired: 5 in, 1 out]
                n158 = case shown="No Error" w197 {
                  tunnel: w202 -> [w207 w225]
                  tunnel: w201 -> [w206 _]
                  tunnel: w199 -> [w204 _]
                  tunnel: w196 -> [w203 _]
                  frame No Error {
                    n159 = Strip Path(path=w204) -> (name=w205:string)  [unwired: 1 out]
                    n160 = case "Load File?" shown="False" w207 {
                      tunnel: w206 -> [w221 _]
                      tunnel: w205 -> [w215 _]
                      tunnel: w204 -> [w216 _]
                      tunnel: w203 -> [w209 _]
                      frame False {
                        n161 = control-ref of="ListOfBases_Data"() -> (w208:refnum<vi>)
                        n162 = call "PrepareSignals.vi"("ListOfBases_Data"=w208, "SetValueInfo in"=w209, "setfile path"=w216, "Enum"=enum16{"Save", "Load"}."Load", "Display Message to \nUser"=TRUE ("Display Message to \nUser"), "DIMControSet in"=w221) -> ("indexed loaded Array"=w219:dbl[][], "Name Array"=w218:string[], "DIMControSet out"=w220:refnum<vi>[])  [unwired: 3 in]
                        n163 = call "CompareArrays.vi"("indexed loaded Array"=w219, "Name Array"=w218, "DIMControSet"=w220) -> ("Table for loading values"=w217:string[][])  [unwired: 4 in]
                        n164 = call "LoadSet.vi"("File Name In"=w215, "output array"=w217) -> ("File Name out"=w214:string, "Accepted"=w213:bool)  [unwired: 8 in]
                        n165 = case "Accepted?" shown="True" w213 {
                          tunnel: w214 -> [_ w224]
                          tunnel: "ionguide" ("string") -> [_ w223]
                          frame False {
                          }
                          frame True {
                            n166 = call "UpdateLastLoadedFile.vi"("LoadOrSave"=enum16{"Load", "Save"}."Load", "GUIName"=w223, "FileNameIn"=w224) -> ()  [unwired: 13 in]
                          }
                        }
                      }
                      frame True {
                      }
                    }
                  }
                  frame Error {
                    n167 = Not(x=w225) -> (.not. x?=w226:bool)
                    n168 = call "Display Message to User"("Enable"=w226) -> ()  [unwired: 9 in, 2 out]
                  }
                }
              }
              frame "BUNAPP_FILE_ZERO" {
                w232 = "All Signals Go To Zero.set" ("File Name")
                # "Set Voltages to Zero"
                n169 = property on="SetFileLocation" class="Path"() -> ("Value"=w230:path)  [unwired: 2 in, 2 out]
                n170 = Build Path(base path=w230, name or relative path=w232) -> (appended path=w231:path)
                n171 = control-ref of="ListOfBases_Data"() -> (w227:refnum<vi>)
                n172 = call "PrepareSignals.vi"("ListOfBases_Data"=w227, "SetValueInfo in"=w228, "setfile path"=w231, "Enum"=enum16{"Save", "Load"}."Load", "Display Message to \nUser"=TRUE ("Display Message to \nUser"), "DIMControSet in"=w241) -> ("indexed loaded Array"=w239:dbl[][], "Name Array"=w238:string[], "DIMControSet out"=w240:refnum<vi>[])  [unwired: 3 in]
                n173 = call "CompareArrays.vi"("indexed loaded Array"=w239, "Name Array"=w238, "DIMControSet"=w240) -> ("Table for loading values"=w237:string[][])  [unwired: 4 in]
                n174 = call "LoadSet.vi"("File Name In"=w232, "output array"=w237) -> ("File Name out"=w235:string, "Accepted"=w236:bool)  [unwired: 8 in]
                n175 = case "Accepted?" shown="True" w236 {
                  tunnel: w235 -> [_ w244]
                  tunnel: "ionguide" ("string") -> [_ w243]
                  frame False {
                  }
                  frame True {
                    n176 = call "UpdateLastLoadedFile.vi"("LoadOrSave"=enum16{"Load", "Save"}."Load", "GUIName"=w243, "FileNameIn"=w244) -> ()  [unwired: 13 in]
                  }
                }
              }
              frame "Legend" {
                # "Open Legend"
                n177 = call "Legend.vi"("i ref in"=refnum<vi> refnum) -> ("i ref out"=→"i ref out":refnum<vi>)  [unwired: 10 in]
              }
              frame "Delayed DC" {
                # "Open Front Panel"
                # "Start VI"
                # "Call vit"
                # "Open Delayed DC VI"
                n178 = Open VI Reference(vi path=path "DelayedDC.vit", options=8) -> (vi reference=w253:refnum<vi>, error out=w252:errorcluster)  [unwired: 4 in]
                n179 = invoke class="VI" method="Run VI"(reference=w253, error in=w252, "Wait until done"=FALSE ("Wait Until Done"), "Auto Dispose Ref"=TRUE ("Auto Dispose Reference")) -> (reference out=w248:refnum<vi>, error out=w247:errorcluster)  [unwired: 1 in, 3 out]
                n180 = invoke class="VI" method="FP.Open"(reference=w248, error in=w247, "Activate"=TRUE ("Activate?")) -> (reference out=→"vi reference":refnum<vi>, error out=→"error out":errorcluster)  [unwired: 2 in, 3 out]
              }
              frame "BUNAPP_FILE_EXIT" {
                # "Exit"
              }
            }
          }
          event Value Change {
            n181 = event-data() -> ("NewVal"=w262:T1)  [unwired: 1 in]
            n182 = stacked-sequence "Update Set File Location and Last Loaded File" {
              tunnel: w262 -> [w264 _]
              tunnel: w261 -> [_ w286]
              tunnel: w259 -> [_ w281]
              frame #0 {
                # "Update Set File Location"
                n183 = Unbundle By Name(w264) -> ("data"=w273:string, "no link"=w272:bool, "quality"=w271:i32)
                n184 = case "Link?" shown="False" w272 {
                  tunnel: w271 -> [w277 _]
                  tunnel: [w276 UtilityLib.valueStatus."no info available" ("valueStatus")] -> w274
                  tunnel: w273 -> [w275 _]
                  tunnel: [w275 w278] -> w269
                  frame False {
                    n185 = call "CoreLib.quality 2 status.vi"("quality"=w277) -> ("valueStatus"=w276:T7)  [unwired: 18 in]
                  }
                  frame True {
                    n186 = call "EmptyString.vi"() -> ("String"=w278:string)
                  }
                }
                n187 = Type Cast(type="" ("regular expression"), x=w269) -> (*(type *) &x=w268:string)
                n188 = String To Path(string=w268) -> (path=w265:path)
                n189 = control-ref of="SetFileLocation"() -> (w263:refnum<vi>)
                n190 = Build Path(base path=w265, name or relative path="IonGuideControl") -> (appended path=w266:path)
                n191 = property class="Path"(reference=w263, "Value"=w266) -> ()  [unwired: 1 in, 2 out]
                n192 = call "UtilityLib.set color of GUI object.vi"("GUI object Ref"=w263, "valueStatus"=w274) -> ()  [unwired: 17 in, 1 out]
              }
              frame #1 {
                # "Update Last Loaded File"
                n193 = control-ref of="SetFileLocation"() -> (w285:refnum<vi>)
                n194 = control-ref of="Last Loaded File"() -> (w284:refnum<vi>)
                n195 = control-ref of="Last Loaded File_Data"() -> (w282:refnum<vi>)
                n196 = control-ref of="ListOfBases_Data"() -> (w280:refnum<vi>)
                n197 = property class="Clust (strict)"(reference=w282) -> ("Value"=w287:T8)  [unwired: 1 in, 2 out]
                n198 = call "LastLoadedFile.vi"("SetFileLocation"=w285, "Last Loaded File"=w284, "GUIName"="ionguide", "DIMControSet in"=w286, "SetValueInfo in"=w281, "NewVal"=w287, "ListOfBases_Data"=w280) -> ()  [unwired: 13 in]
              }
            }
          }
          event Value Change {
            # "Update Last Loaded File"
            n199 = event-data() -> ("NewVal"=w292:T1)  [unwired: 1 in]
            n200 = control-ref of="SetFileLocation"() -> (w291:refnum<vi>)
            n201 = control-ref of="Last Loaded File"() -> (w290:refnum<vi>)
            n202 = control-ref of="ListOfBases_Data"() -> (w288:refnum<vi>)
            n203 = call "LastLoadedFile.vi"("SetFileLocation"=w291, "Last Loaded File"=w290, "GUIName"="ionguide", "DIMControSet in"=w293, "SetValueInfo in"=w289, "NewVal"=w292, "ListOfBases_Data"=w288) -> ()  [unwired: 13 in]
          }
          event "IonGuideBase": Value Change {
            w296 = "IonGuideBase" ("string")
            # "Update  Set Values"
            n204 = event-data() -> ("NewVal"=w299:dbl, "OldVal"=w298:dbl)  [unwired: 1 in, 4 out]
            n205 = control-ref of="ListOfBases_Data"() -> (w297:refnum<vi>)
            n206 = call "IsBaseInRange.vi"("SetValueInfo"=w304, "DIMControSet"=w303, "ListOfBases_Data"=w297, "NewVal in"=w299, "Base Name"=w296) -> ("NewVal Out"=w300:dbl, "In Range"=w301:bool)  [unwired: 13 in]
            n207 = case "Base In Range?" shown="True" w301 {
              tunnel: w300 -> [_ w309]
              tunnel: w298 -> [w305 _]
              tunnel: w296 -> [_ w306]
              frame False {
                n208 = property on="IonGuideBase" class="DigNum (strict)"("Value"=w305) -> ()  [unwired: 2 in, 2 out]
              }
              frame True {
                n209 = call-poly "CoreLib.data 2 byte array.vi"("i16"=i16 0 ("element")) -> ("byteArray out"=w308:T6)  [unwired: 18 in]
                n210 = property on="IonGuideBase" class="DigNum (strict)"("Value"=w309) -> ()  [unwired: 2 in, 2 out]
                n211 = call-poly "CoreLib.data 2 byte array.vi"("byteArray"=w308, "f64"=w309) -> ("byteArray out"=w313:T6)  [unwired: 17 in]
                n212 = Flatten To String(anything=TRUE) -> (data string=w312:string)  [unwired: 3 in, 2 out]
                n213 = Concatenate Strings("SetPLC" ("string"), w306) -> (w318:string)
                n214 = call-poly "CoreLib.data 2 byte array.vi"("byteArray"=w313, "string"=w312) -> ("byteArray out"=w310:T6)  [unwired: 17 in]
                n215 = Bundle By Name(cluster="call cluster in", "Object"="PLC", "Selector"=w318, "CallType"=enum16{"simple", "synchronous", "asynchronous"}."simple", "Data"=w310) -> (w315:T4)
                n216 = call "CoreLib.call process.vi"("call cluster in"=w315) -> ()  [unwired: 13 in, 2 out]
              }
            }
          }
          event Value Change {
            # "Update TestBase1 Set Value"
            n217 = event-data() -> ("CtlRef"=w323:refnum<vi>, "NewVal"=w327:T2)  [unwired: 1 in, 4 out]
            n218 = Unbundle By Name(w327) -> ("data"=w328:dbl[], "no link"=w329:bool, "quality"=w331:i32)
            n219 = property on="FileUpToDate" class="Bool (strict)"() -> ("Value"=w320:bool)  [unwired: 2 in, 2 out]
            n220 = case "Link?" shown="True" w329 {
              tunnel: w331 -> [w333 _]
              tunnel: [w332 UtilityLib.valueStatus."no info available" ("valueStatus")] -> w330
              tunnel: w328 -> [w335 _]
              tunnel: [w334 inf] -> w324
              frame False {
                n221 = call "CoreLib.quality 2 status.vi"("quality"=w333) -> ("valueStatus"=w332:T7)  [unwired: 18 in]
                n222 = Index Array(array=w335, index #1=0 ("index")) -> (element #1=w334:dbl)  [unwired: 1 in, 1 out]
              }
              frame True {
              }
            }
            n223 = call "FileUpToDate.vi"("FileUpToDate in"=w320, "DIMControSet out"=w322, "CtlRef"=w323) -> ("FileUpToDate out"=w321:bool)  [unwired: 16 in]
            n224 = property on="FileUpToDate" class="Bool (strict)"("Value"=w321) -> ()  [unwired: 2 in, 2 out]
            n225 = control-ref of="IonGuideBase"() -> (w326:refnum<vi>)
            n226 = property on="IonGuideBase" class="DigNum (strict)"("Value"=w324) -> ()  [unwired: 2 in, 2 out]
            n227 = call "UtilityLib.set color of GUI object.vi"("GUI object Ref"=w326, "valueStatus"=w330) -> ()  [unwired: 17 in, 1 out]
          }
          event Value Change {
            # "Find Monitor Value Index"
            # "Updating a Monitor Value"
            n228 = event-data() -> ("CtlRef"=w342:refnum<vi>, "NewVal"=w346:T3)  [unwired: 1 in, 4 out]
            n229 = Search 1D Array(1D array=w343, element=w342) -> (index of element=w344:i32)  [unwired: 1 in]
            n230 = Index Array(array=w339, index=w344) -> (element=w340:refnum<vi>)
            n231 = Not A Number/Path/Refnum?(number/path/refnum=w340) -> (NaN/Path/Refnum?=w341:bool)
            n232 = case "Indicator does not exists?" shown="False" w341 {
              tunnel: w346 -> [_ w353]
              tunnel: w340 -> [_ w347]
              frame True {
              }
              frame False {
                n233 = Unbundle By Name(w353) -> ("data"=w349:dbl, "no link"=w350:bool, "quality"=w352:i32)
                n234 = case shown="False" w350 {
                  tunnel: w352 -> [w356 _]
                  tunnel: [w355 UtilityLib.valueStatus."no info available" ("valueStatus")] -> w351
                  tunnel: w349 -> [w354 _]
                  tunnel: [w354 inf] -> w348
                  frame False {
                    n235 = call "CoreLib.quality 2 status.vi"("quality"=w356) -> ("valueStatus"=w355:T7)  [unwired: 18 in]
                  }
                  frame True {
                  }
                }
                n236 = property class="DigNum (strict)"(reference=w347, "Value"=w348) -> ()  [unwired: 1 in, 2 out]
                n237 = call "TextColor.vi"("valueStatus"=w351, "reference"=w347) -> ()  [unwired: 10 in]
              }
            }
          }
          event Value Change {
            n238 = event-data() -> ("CtlRef"=w360:refnum<vi>)  [unwired: 1 in, 5 out]
            n239 = property on="FileUpToDate" class="Bool (strict)"() -> ("Value"=w359:bool)  [unwired: 2 in, 2 out]
            n240 = call "FileUpToDate.vi"("FileUpToDate in"=w359, "DIMControSet out"=w361, "CtlRef"=w360) -> ("FileUpToDate out"=w362:bool)  [unwired: 16 in]
            n241 = property on="FileUpToDate" class="Bool (strict)"("Value"=w362) -> ()  [unwired: 2 in, 2 out]
          }
          event "IGADC1", "IGADC3", "uPlate1", "IGADC2", "RFamp1", "uDC2", "uDC1", "uPlate2", "RFamp2", "DC4", "DC5", "RFphase1", "RFphase2", "RFamp3", "Mass", "Offset", "Alpha", "DC7", "DC6", "DC8": Value Change {
            # "Find sub-panel index"
            # "opening or closing a sub-panel"
            n242 = event-data() -> ("CtlRef"=w364:refnum<vi>)  [unwired: 1 in, 3 out]
            n243 = Search 1D Array(1D array=w365, element=w364) -> (index of element=w370:i32)  [unwired: 1 in]
            n244 = Index Array(array=w371, index=w370) -> (element=w368:refnum<vi>)
            n245 = invoke class="Bool" method="Reinit To Default"(reference=w364) -> ()  [unwired: 2 in, 3 out]
            n246 = property class="VI"(reference=w368) -> ("Front Panel.Open"=w367:bool)  [unwired: 1 in, 2 out]
            n247 = case "Panel Already Open?" shown="False" w367 {
              tunnel: w364 -> [w373 _]
              tunnel: w368 -> [_ w375]
              tunnel: [w372 refnum<vi> refnum ("vi reference")] -> w366
              frame False {
                n248 = call "OpenPanel.vi"("CtlRef"=w373) -> ("vi reference"=w372:refnum<vi>)  [unwired: 2 in]
              }
              frame True {
                n249 = call "PanelClose.vi"("vi reference"=w375) -> ()
              }
            }
            n250 = Replace Array Subset(array=w371, new element=w366, index=w370) -> (w369:refnum<vi>[])
          }
          event "Close All Panels": Value Change {
            n251 = event-data() -> ()  [unwired: 1 in, 6 out]
            n252 = case "Close Open Panels?" shown="False" "Close All Panels" {
              tunnel: w378 -> [w379 w381]
              tunnel: [w379 w380] -> w376
              frame False {
              }
              frame True {
                n253 = for "Close Open Panels" {
                  tunnel: w381 -> [w383] mode=indexing
                  tunnel: w381 -> [w382]
                  tunnel: [w382] -> w380
                  n254 = call "PanelClose.vi"("vi reference"=w383) -> ()
                }
              }
            }
          }
          event Timeout {
            # "Timeout"
            n255 = event-data() -> ()  [unwired: 1 in, 3 out]
          }
          event Panel Close? {
            n256 = event-data() -> ()  [unwired: 1 in, 4 out]
            n257 = stacked-sequence {
              tunnel: w388 -> [w395 _]
              tunnel: w387 -> [w394 _]
              tunnel: w386 -> [w393 _]
              tunnel: w385 -> [w396 _]
              frame #0 {
                # "Release DIM Services"
                n258 = for "Close Open Panels" {
                  tunnel: w396 -> [w406] mode=indexing
                  n259 = call "PanelClose.vi"("vi reference"=w406) -> ()
                }
                n260 = for "For Each Service" {
                  tunnel: w395 -> [w404] mode=indexing
                  n261 = Not A Number/Path/Refnum?(number/path/refnum=w404) -> (NaN/Path/Refnum?=w403:bool)
                  n262 = case "Not a Reference?" shown="False" w403 {
                    tunnel: w404 -> [w405 _]
                    frame False {
                      n263 = call "DimIndicators.dic_release_service.vi"("controlRef"=w405) -> ()  [unwired: 18 in, 1 out]
                    }
                    frame True {
                    }
                  }
                }
                n264 = for "For Each Service" {
                  tunnel: w394 -> [w401] mode=indexing
                  n265 = Not A Number/Path/Refnum?(number/path/refnum=w401) -> (NaN/Path/Refnum?=w400:bool)
                  n266 = case "Not a Reference?" shown="False" w400 {
                    tunnel: w401 -> [w402 _]
                    frame False {
                      n267 = call "DimIndicators.dic_release_service.vi"("controlRef"=w402) -> ()  [unwired: 18 in, 1 out]
                    }
                    frame True {
                    }
                  }
                }
                n268 = for "For Each Service" {
                  tunnel: w393 -> [w398] mode=indexing
                  n269 = Not A Number/Path/Refnum?(number/path/refnum=w398) -> (NaN/Path/Refnum?=w397:bool)
                  n270 = case "Not a Reference?" shown="False" w397 {
                    tunnel: w398 -> [w399 _]
                    frame False {
                      n271 = call "DimIndicators.dic_release_service.vi"("controlRef"=w399) -> ()  [unwired: 18 in, 1 out]
                    }
                    frame True {
                    }
                  }
                }
                n272 = control-ref of="ListOfBases_Data"() -> (w390:refnum<vi>)
                n273 = control-ref of="SetFileLocation_Data"() -> (w391:refnum<vi>)
                n274 = control-ref of="Last Loaded File_Data"() -> (w392:refnum<vi>)
                n275 = call "DimIndicators.dic_release_service.vi"("controlRef"=w390) -> ()  [unwired: 18 in, 1 out]
                n276 = call "DimIndicators.dic_release_service.vi"("controlRef"=w391) -> ()  [unwired: 18 in, 1 out]
                n277 = call "DimIndicators.dic_release_service.vi"("controlRef"=w392) -> ()  [unwired: 18 in, 1 out]
              }
              frame #1 {
                # "Close Front Panel"
                n278 = Current VI's Path() -> (path=w410:path)
                n279 = Open VI Reference(vi path=w410) -> (vi reference=w408:refnum<vi>, error out=w407:errorcluster)  [unwired: 5 in]
                n280 = property class="VI"(reference=w408, error in=w407, "Front Panel Window:Open"=FALSE) -> ()  [unwired: 2 out]
              }
            }
            n281 = event-data() -> ()  [unwired: 2 in, 1 out]
          }
        }
      }
    }
    frame #8 {
      n282 = stacked-sequence {
        tunnel: w414 -> [w417 _ _]
        tunnel: w413 -> [w421 _ _]
        tunnel: w412 -> [w418 _ _]
        tunnel: w411 -> [w419 _ _]
        frame #0 {
          # "Release DIM Services"
          n283 = control-ref of="ListOfBases_Data"() -> (w415:refnum<vi>)
          n284 = control-ref of="Last Loaded File_Data"() -> (w420:refnum<vi>)
          n285 = control-ref of="SetFileLocation_Data"() -> (w416:refnum<vi>)
          n286 = call "DimIndicators.dic_release_service.vi"("controlRef"=w415) -> ()  [unwired: 18 in, 1 out]
          n287 = call "DimIndicators.dic_release_service.vi"("controlRef"=w420) -> ()  [unwired: 18 in, 1 out]
          n288 = call "DimIndicators.dic_release_service.vi"("controlRef"=w416) -> ()  [unwired: 18 in, 1 out]
          n289 = for "For Each Service" {
            tunnel: [w428] -> _ mode=indexing
            tunnel: w419 -> [w428] mode=indexing
            n290 = Not A Number/Path/Refnum?(number/path/refnum=w428) -> (NaN/Path/Refnum?=w429:bool)
            n291 = case "Not a Reference?" shown="False" w429 {
              tunnel: w428 -> [w430 _]
              frame False {
                n292 = call "DimIndicators.dic_release_service.vi"("controlRef"=w430) -> ()  [unwired: 18 in, 1 out]
              }
              frame True {
              }
            }
          }
          n293 = for "For Each Service" {
            tunnel: w418 -> [w425] mode=indexing
            tunnel: [w425] -> _ mode=indexing
            n294 = Not A Number/Path/Refnum?(number/path/refnum=w425) -> (NaN/Path/Refnum?=w426:bool)
            n295 = case "Not a Reference?" shown="False" w426 {
              tunnel: w425 -> [w427 _]
              frame False {
                n296 = call "DimIndicators.dic_release_service.vi"("controlRef"=w427) -> ()  [unwired: 18 in, 1 out]
              }
              frame True {
              }
            }
          }
          n297 = for "For Each Service" {
            tunnel: w417 -> [w422] mode=indexing
            tunnel: [w422] -> _ mode=indexing
            n298 = Not A Number/Path/Refnum?(number/path/refnum=w422) -> (NaN/Path/Refnum?=w423:bool)
            n299 = case "Not a Reference?" shown="False" w423 {
              tunnel: w422 -> [w424 _]
              frame False {
                n300 = call "DimIndicators.dic_release_service.vi"("controlRef"=w424) -> ()  [unwired: 18 in, 1 out]
              }
              frame True {
              }
            }
          }
          n301 = for "Close Open Panels" {
            tunnel: w421 -> [w431] mode=indexing
            n302 = call "PanelClose.vi"("vi reference"=w431) -> ()
          }
        }
        frame #1 {
          # "Close Front Panel"
          n303 = Current VI's Path() -> (path=w435:path)
          n304 = Open VI Reference(vi path=w435) -> (vi reference=w433:refnum<vi>, error out=w432:errorcluster)  [unwired: 5 in]
          n305 = property class="VI"(reference=w433, error in=w432, "Front Panel Window:Open"=FALSE) -> ()  [unwired: 2 out]
        }
        frame #2 {
          # "Stop Panel"
          n306 = Stop(stop? (T)=TRUE) -> ()
        }
      }
    }
  }
  n307 = call "LVDimInterface.dim_operate.vi"("DNSNode"="lebit-balcony" ("DNS node")) -> ()  [unwired: 19 in]
